vi "GetSheredData.vi"(0 "reference in":refnum<class "GUI.lvclass">, 11 "error in (no error)":errorcluster) -> (4 "reference out":refnum<class "GUI.lvclass">, 6 "data":T1, 15 "error out":errorcluster)   [LabVIEW 2019, in "GUI.lvclass"]
uses:
  GUI.lvclass
  Shered Data.ctl
  WindowsState.ctl
  GUI.lvclass/GUI.ctl
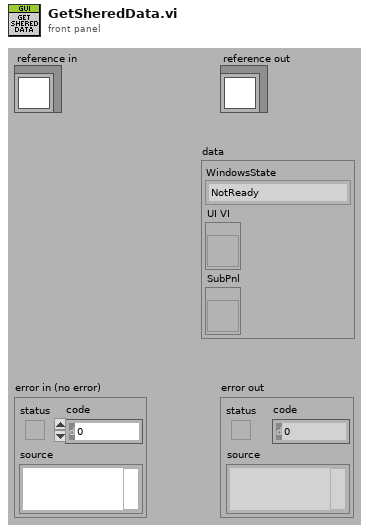
[diagram p1: front panel]
types:
  T1 = typedef "GUI.lvclass/Shered Data.ctl" = cluster{"WindowsState":T2, "UI VI":refnum<vi>, "SubPnl":refnum<vi>}
  T2 = typedef "GUI.lvclass/WindowsState.ctl" = enum16{"NotReady", "Ready", "Inserted", "Opened"}
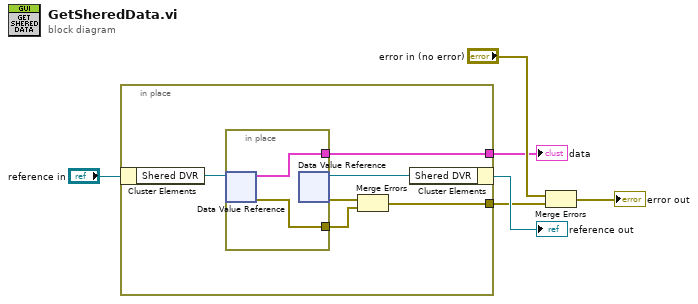
[diagram p0: block diagram]
diagram:
  n1 = in-place {
    in-place-border: [w8] -> w4
    in-place-border: [w7] -> w1
    n2 = in-place-cluster #1("reference in") -> ("Shered DVR"=w12:refnum<data-value>)
    n3 = in-place {
      in-place-border: [w14] -> w9
      in-place-border: [w13] -> w7
      n4 = in-place-dvr #2(w12) -> (w13:T1, w14:errorcluster)
      n5 = in-place-dvr #2() -> (w11:refnum<data-value>, w10:errorcluster)  [unwired: 1 in]
    }
    n6 = Merge Errors(w10, w9) -> (w8:errorcluster)
    n7 = in-place-cluster #1("Shered DVR"=w11) -> (→"reference out":refnum<class "GUI.lvclass">)
  }
  "data" <- w1
  n8 = Merge Errors("error in (no error)", w4) -> (→"error out":errorcluster)
